vi "GET USER ID.vi"(11 "BYU ID IN":string) -> (3 "USER/ITEM DATA TRANSFER":T1(array[cluster]))   [LabVIEW 2019]
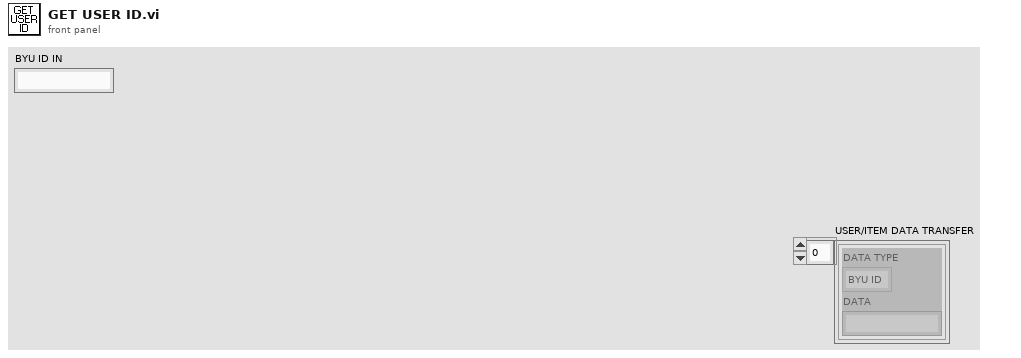
[diagram p1: front panel]
types:
  T1 = cluster{"DATA TYPE":enum16{"BYU ID", "ME#/IDENTIFIER", "BYU ICN"}, "DATA":string}[]
  T2 = cluster{"DATA TYPE":enum16{"BYU ID", "ME#/IDENTIFIER", "BYU ICN"}, "DATA":string}
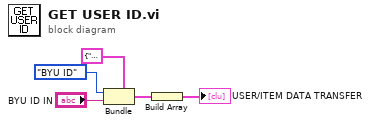
[diagram p0: block diagram]
diagram:
  n1 = Bundle(cluster=T2 {"DATA TYPE"=enum."BYU ID", "DATA"=""} ("USER/ITEM DATA TRANSFER"), "DATA TYPE"=enum16{"BYU ID", "ME#/IDENTIFIER", "BYU ICN"}."BYU ID", "DATA"="BYU ID IN") -> (w3:T2)
  n2 = Build Array(w3) -> (→"USER/ITEM DATA TRANSFER":T1)
